vi "Парсер_Сложность.vi"() -> ()   [LabVIEW 2018]
uses:
  <vilib>/Utility/file.llb/Read Delimited Spreadsheet (string).vi
panel:
  out "Текущая строка":i32
  in  "Строка":bool
  in  "Стоп":bool
  out "Массив":string[](array[string])=["0", "1", "0", "0", "0", "0", "0", "0", "0", "0", "0", "0", "0", "0", "0", "0", "1", "0", "0", "0", "0", "0", "0", "1", "1", "1", "1", "0", "0", "0", "0", "0", "0", "0", "1", "1", "1", "1", "1", "1", "1", "0", "0", "0", "0", "0", "0", "0", "1", "1", "1", "1", "1", "1", "1", "0", "0", "0", "0", "0", "0", "0", "1", "1", "1", "1", "1", "1", "1", "0", "0", "0", "0", "0", "0", "0", "1", "1", "1", "1", "1", "1", "1", "X", "X", "X", "X", "X", "X", "X", "X", "X", "X", "X", "X", "X", "X", "X", "X", "X", "X", "X", "X", "X", "X", "X", "X", "X", "X", "X", "X", "X", "X", "X", "X", "X", "X", "X", "X", "X"]
  in  "Все строки":string[][](array[string])=array496131x1[496131 elements]
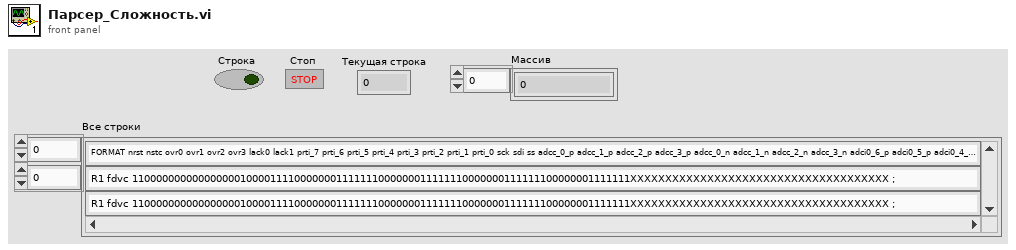
[diagram p1: front panel]
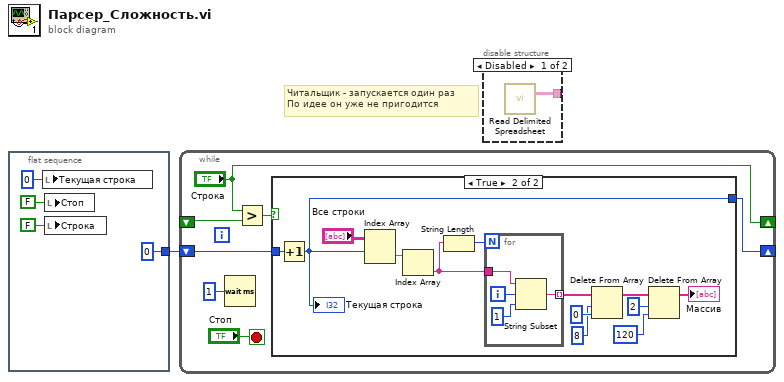
[diagram p0: block diagram]
diagram:
  # "Читальщик - запускается один раз\nПо идее он уже не пригодится"
  n1 = flat-sequence {
    tunnel: [0] -> w1
    frame #0 {
      n2 = local write "Текущая строка"(0 ("Текущая строка")) -> ()
      n3 = local write "Стоп"(FALSE ("Стоп")) -> ()
      n4 = local write "Строка"(FALSE ("Строка")) -> ()
    }
  }
  n5 = while {
    shift-right: [w11] -> _
    shift-left: w1 -> [w12]
    shift-right: ["Строка"] -> _
    shift-left: _ -> [w7]
    stop <- "Стоп" stop-if-true
    n6 = Wait (ms)(milliseconds to wait=u32 1) -> ()  [unwired: 1 out]
    n7 = Greater?(x="Строка", y=w7) -> (0:w9:bool)
    n8 = case shown="True" w9 {
      tunnel: w12 -> [w13 w26]
      tunnel: [w13 w25] -> w11
      frame False {
      }
      frame True {
        n9 = Increment(x=w26) -> (x+1=w25:i32)
        "Текущая строка" <- w25
        n10 = Index Array(array="Все строки", index (row)=w25) -> (element=w23:string[])  [unwired: 1 in]
        n11 = Index Array(array=w23) -> (element=w21:string)  [unwired: 1 in]
        n12 = String Length(string=w21) -> (length=w22:i32)
        n13 = for {
          N: w22 -> [_]
          tunnel: w21 -> [w30]
          tunnel: [w27] -> w20 mode=indexing
          i -> [w29]
          n14 = String Subset(string=w30, offset (0)=w29, length (rest)=1 ("length (rest)")) -> (substring=w27:string)
        }
        n15 = Delete From Array(array=w20, length=8, index=0) -> (array with subset deleted=w19:string[])  [unwired: 1 out]
        n16 = Delete From Array(array=w19, length=2, index=120) -> (array with subset deleted=→"Массив":string[])  [unwired: 1 out]
      }
    }
  }
  n17 = disable-structure shown="Disabled" {
    disable-tunnel: [w31 _] -> _
    frame Disabled {
      n18 = call-poly <vilib>:"Read Delimited Spreadsheet.vi"() -> ("all rows"=w31:string[][])  [unwired: 10 in, 5 out]
    }
    frame Enabled {
    }
  }
